vi "TEMPLATE.vi"(6 "Teller":refnum<class "Teller.lvclass">, 8 "Error in":errorcluster, 11 "TEMPLATE in":refnum<class "TEMPLATE jettl Msg.lvclass">) -> (0 "Error out":errorcluster, 3 "TEMPLATE out":refnum<class "TEMPLATE jettl Msg.lvclass">)   [LabVIEW 2025, in "_Template.lvlib" / "Templates.lvlib" / "TEMPLATE jettl Msg.lvlib" / "TEMPLATE jettl Msg.lvclass"]
uses:
  TEMPLATE jettl Msg.lvclass
  jettl/jettl/Teller/Teller.lvclass
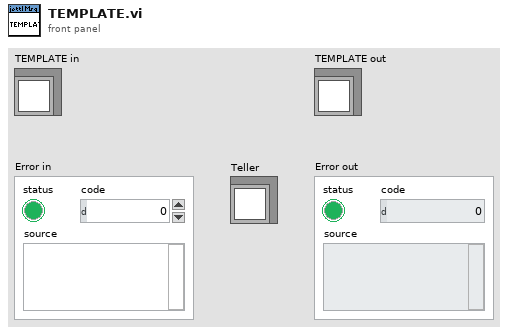
[diagram p1: front panel]
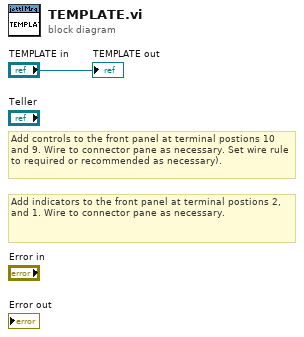
[diagram p0: block diagram]
diagram:
  # "Add indicators to the front panel at terminal postions 2, and 1. Wire to connector pane as necessary."
  # "Add controls to the front panel at terminal postions 10 and 9. Wire to connector pane as necessary. Set wire rule to required or recommended as necessary)."
  "TEMPLATE out" <- "TEMPLATE in"
